vi "stop.vi"(8 "error in (no error)":errorcluster, 9 "CameraSettings":refnum<class "CamaraSettings.lvclass">, 10 "stop":bool, 11 "NetworkPixelfly in":refnum<class "Network_ProEm_WinX32.lvclass">) -> (0 "error out":errorcluster, 1 "imageSaved":bool, 2 "stopped?":bool, 3 "NetworkPixelfly out":refnum<class "Network_ProEm_WinX32.lvclass">)   [LabVIEW 2011, in "Hardware.lvlib" / "HWControllers.lvlib" / "Network_ProEm_WinX32.lvclass"]
uses:
  Network_ProEm_WinX32.lvclass
  Tools/CameraSettings/CamaraSettings.lvclass
  Channels/Camera/Camera/Camera.lvclass
  NetworkCamera.lvclass
panel:
  out "ImagesTaken in":i32
  out "ImagesTaken":i32
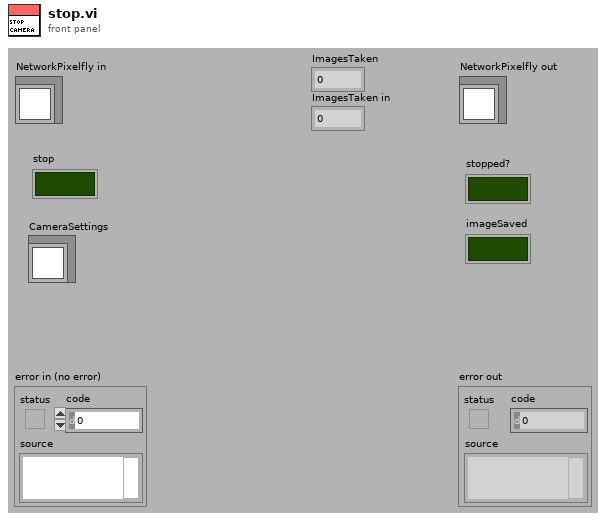
[diagram p1: front panel]
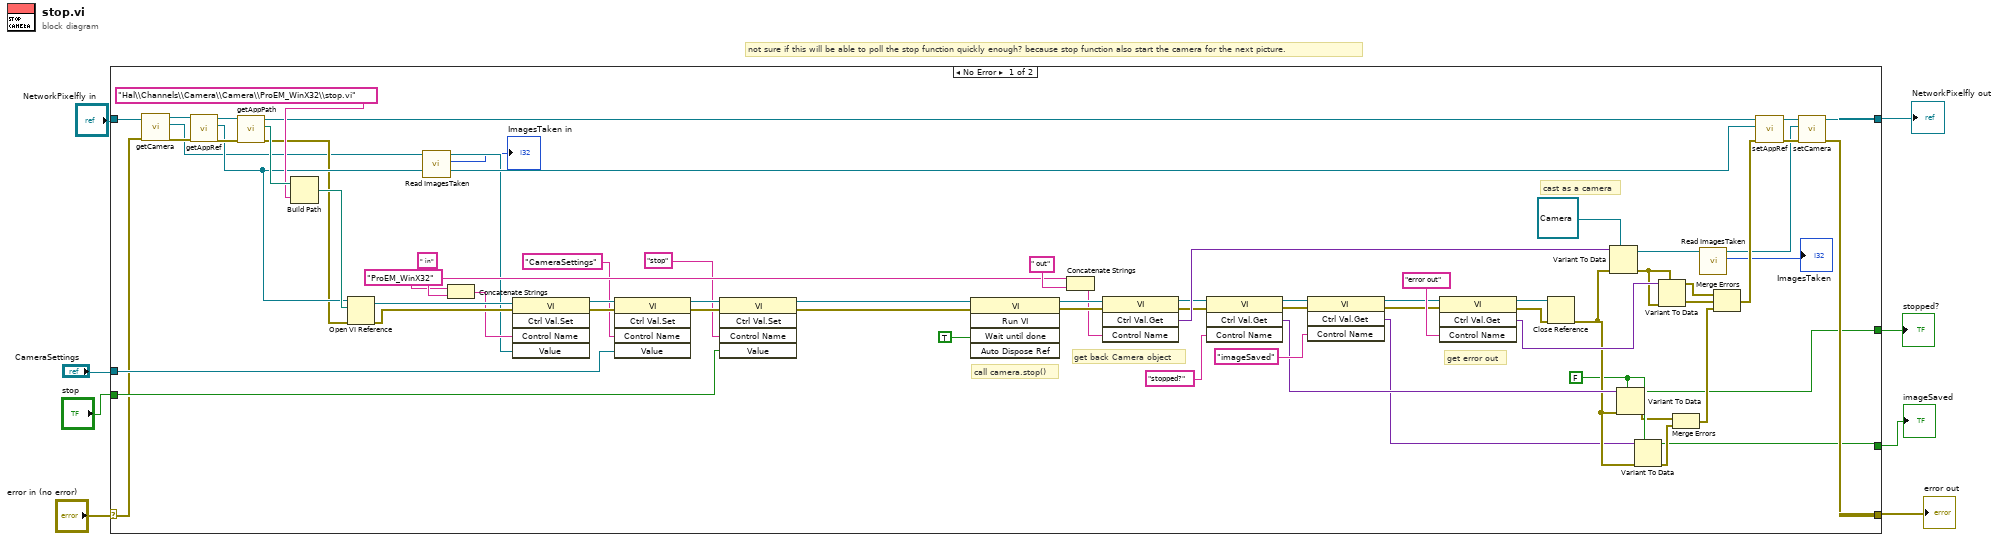
[diagram p0: block diagram]
diagram:
  # "not sure if this will be able to poll the stop function quickly enough? because stop function also start the camera for the next picture."
  n1 = case shown="No Error" "error in (no error)" {
    selector: "error in (no error)" -> [w35 w79]
    tunnel: [w52 w79] -> w6
    tunnel: [w55 w78] -> w7
    tunnel: "NetworkPixelfly in" -> [w61 w78]
    tunnel: "CameraSettings" -> [w46 _]
    tunnel: "stop" -> [w44 _]
    tunnel: [w18 _] -> w2
    tunnel: [w17 _] -> w1
    frame No Error {
      w22 = FALSE
      w58 = "ProEM_WinX32" ("Control name")
      # "get error out"
      # "get back Camera object"
      # "call camera.stop()"
      # "cast as a camera"
      n2 = call "getCamera.vi"("error in (no error)"=w35, "NetworkCamera in"=w61) -> ("error out"=w64:errorcluster, "Camera"=w11:refnum<class "Camera.lvclass">, "NetworkCamera out"=w65:refnum<class "Network_ProEm_WinX32.lvclass">)  [unwired: 7 in]
      n3 = call "getAppRef.vi"("error in (no error)"=w64, "NetworkCamera in"=w65) -> ("error out"=w62:errorcluster, "appRef"=w54:refnum<vi>, "NetworkCamera out"=w63:refnum<class "Network_ProEm_WinX32.lvclass">)  [unwired: 7 in]
      n4 = call "getAppPath.vi"("error in (no error)"=w62, "NetworkCamera in"=w63) -> ("error out"=w34:errorcluster, "appPath"=w60:path, "NetworkCamera out"=w57:refnum<class "Network_ProEm_WinX32.lvclass">)  [unwired: 7 in]
      n5 = Build Path(base path=w60, name or relative path="Hal\\Channels\\Camera\\Camera\\ProEM_WinX32\\stop.vi" ("viPath")) -> (appended path=w77:path)
      n6 = Open VI Reference(application reference (local)=w54, vi path=w77, error in (no error)=w34) -> (vi reference=w71:refnum<vi>, error out=w70:errorcluster)  [unwired: 3 in]
      n7 = call "Read ImagesTaken.vi"("Camera in"=w11) -> ("ImagesTaken"=→"ImagesTaken in":i32, "Camera out"=w10:refnum<class "Camera.lvclass">)  [unwired: 8 in, 1 out]
      n8 = Concatenate Strings(w58, " in") -> (w68:string)
      n9 = invoke class="VI" method="Ctrl Val.Set"(reference=w71, error in=w70, "Control Name"=w68, "Value"=w10) -> (reference out=w51:refnum<vi>, error out=w49:errorcluster)  [unwired: 1 in, 3 out]
      n10 = invoke class="VI" method="Ctrl Val.Set"(reference=w51, error in=w49, "Control Name"="CameraSettings", "Value"=w46) -> (reference out=w50:refnum<vi>, error out=w48:errorcluster)  [unwired: 1 in, 3 out]
      n11 = invoke class="VI" method="Ctrl Val.Set"(reference=w50, error in=w48, "Control Name"="stop", "Value"=w44) -> (reference out=w16:refnum<vi>, error out=w15:errorcluster)  [unwired: 1 in, 3 out]
      n12 = invoke class="VI" method="Run VI"(reference=w16, error in=w15, "Wait until done"=TRUE) -> (reference out=w75:refnum<vi>, error out=w74:errorcluster)  [unwired: 2 in, 3 out]
      n13 = Concatenate Strings(w58, " out") -> (w66:string)
      n14 = invoke class="VI" method="Ctrl Val.Get"(reference=w75, error in=w74, "Control Name"=w66) -> (reference out=w33:refnum<vi>, error out=w30:errorcluster, "Get Control Value Variant"=w72:variant)  [unwired: 1 in, 1 out]
      n15 = invoke class="VI" method="Ctrl Val.Get"(reference=w33, error in=w30, "Control Name"="stopped?") -> (reference out=w32:refnum<vi>, error out=w31:errorcluster, "Get Control Value Variant"=w25:variant)  [unwired: 1 in, 1 out]
      n16 = invoke class="VI" method="Ctrl Val.Get"(reference=w32, error in=w31, "Control Name"="imageSaved") -> (reference out=w29:refnum<vi>, error out=w28:errorcluster, "Get Control Value Variant"=w23:variant)  [unwired: 1 in, 1 out]
      n17 = invoke class="VI" method="Ctrl Val.Get"(reference=w29, error in=w28, "Control Name"="error out") -> (reference out=w43:refnum<vi>, error out=w41:errorcluster, "Get Control Value Variant"=w40:variant)  [unwired: 1 in, 1 out]
      n18 = Close Reference(reference=w43, error in (no error)=w41) -> (error out=w24:errorcluster)
      n19 = Variant To Data(error in=w24, type=refnum<class "Camera.lvclass"> refnum ("Camera out"), Variant=w72) -> (data=w14:refnum<class "Camera.lvclass">, error out=w39:errorcluster)
      n20 = Variant To Data(error in=w24, type=w22, Variant=w25) -> (data=w18:bool, error out=w21:errorcluster)
      n21 = Variant To Data(error in=w24, type=w22, Variant=w23) -> (data=w17:bool, error out=w20:errorcluster)
      n22 = Variant To Data(error in=w39, type=w39, Variant=w40) -> (data=w38:errorcluster, error out=w37:errorcluster)
      n23 = Merge Errors(w21, w20) -> (w19:errorcluster)
      n24 = call "Read ImagesTaken.vi"("Camera in"=w14) -> ("ImagesTaken"=→"ImagesTaken":i32, "Camera out"=w13:refnum<class "Camera.lvclass">)  [unwired: 8 in, 1 out]
      n25 = Merge Errors(w38, w37, w19) -> (w36:errorcluster)
      n26 = call "setAppRef.vi"("error in (no error)"=w36, "appRef"=w54, "NetworkCamera in"=w57) -> ("error out"=w53:errorcluster, "NetworkCamera out"=w56:refnum<class "Network_ProEm_WinX32.lvclass">)  [unwired: 7 in]
      n27 = call "setCamera.vi"("error in (no error)"=w53, "Camera"=w13, "NetworkCamera in"=w56) -> ("error out"=w52:errorcluster, "NetworkCamera out"=w55:refnum<class "Network_ProEm_WinX32.lvclass">)  [unwired: 7 in]
    }
    frame Error {
    }
  }
  "error out" <- w6
  "NetworkPixelfly out" <- w7
  "stopped?" <- w2
  "imageSaved" <- w1
